vi "ImageNoiseBlock.vi"(1 "BERLP":sgl, 3 "BERHP":sgl) -> (8 "Low Power Image":T1(plugin-control), 9 "High-Power Image":T1(plugin-control))   [LabVIEW 2022 SP3]
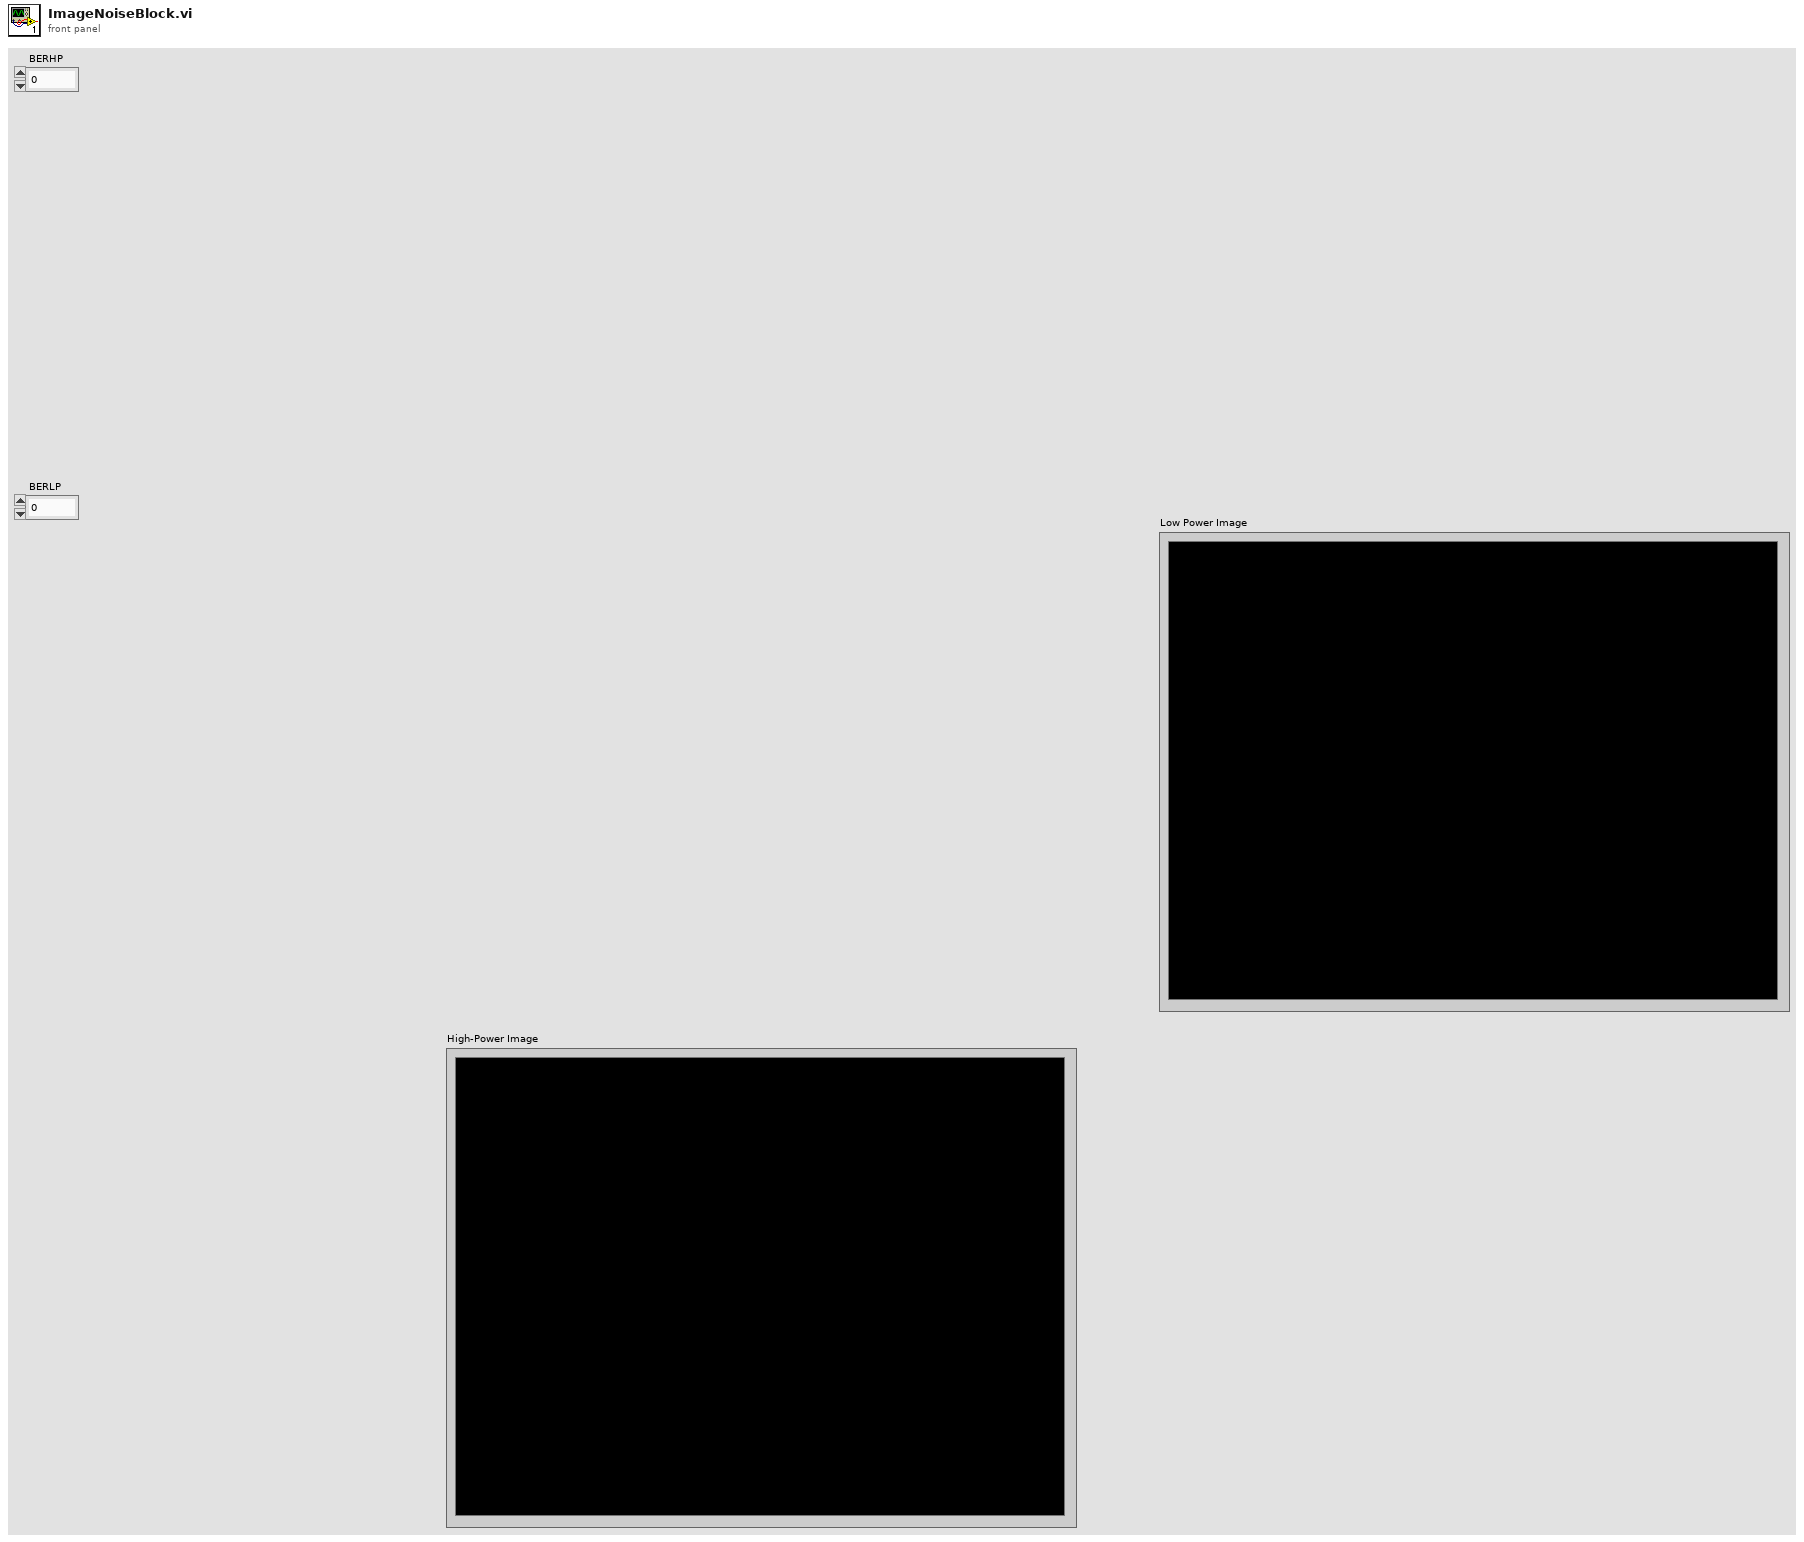
[diagram p1: front panel]
types:
  T1 = typedef "IMAQ Image.ctl" = refnum<image>
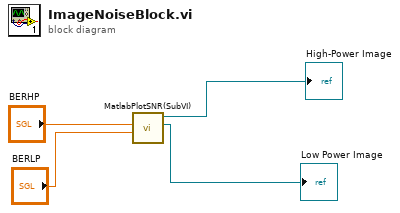
[diagram p0: block diagram]
diagram:
  n1 = call "MatlabPlotSNR(SubVI).vi"("BERLP"="BERLP", "BERHP"="BERHP") -> ("Refnum out LP"=→"Low Power Image":T1, "Refnum out HP"=→"High-Power Image":T1)  [unwired: 8 in]
